vi "TSM Relay Publish Relay Operated.vi"(0 "TSM Relay in":T1={"TSM context"=refnum, "Pin Query Context"=refnum, "TSM Site Numbers"=[], "SSC Relay"=[], "Unfiltered Pins"=[], "Filtered Pins"=[], "Filtered Pins Info"={"Unfiltered Pins Count"=3, "Locations"=[], "Lengths"=[]}}, 1 "Published Data Id":string, 7 "Completed Relay Operations":T5[](array[typedef]) {"Desired State" items=["Open Relay"=20, "Close Relay"=21]}, 11 "error in":errorcluster) -> (4 "TSM Relay out":T1={"TSM context"=refnum, "Pin Query Context"=refnum, "TSM Site Numbers"=[], "SSC Relay"=[], "Unfiltered Pins"=[], "Filtered Pins"=[], "Filtered Pins Info"={"Unfiltered Pins Count"=3, "Locations"=[], "Lengths"=[]}}, 15 "error out":errorcluster)   [LabVIEW 2019]
doc: "This VI publishes the Relay Operated? information from each Relay in the TSM Relay session."
uses:
  SubVIs/TSM SSC Relay.ctl
  <vilib>/NI_TestStand_SemiconductorModule/NI_TestStand_Semiconductor_Module.lvlibp/PinMap/PinQueryContext/MultiplePinMultipleSessionQueryContext/MultiplePinMultipleSessionQueryContext.lvclass
  C:/Program Files/National Instruments/LabVIEW 2019/vi.lib/NI_TestStand_SemiconductorModule/NI_TestStand_Semiconductor_Module.lvlibp/PinMap/PinQueryContext/MultipleSessionPinQueryContext.lvclass
  <vilib>/NI_TestStand_SemiconductorModule/NI_TestStand_Semiconductor_Module.lvlibp/PinMap/General/SemiconductorModuleContext.ctl
  SSC/SSC Relay.ctl
  SubVIs/TSM Filtered Pins Info.ctl
  SubVIs/TSM Relay Completed Operations.ctl
  <instrlib>/niSwitch/niSwitch.llb/niSwitch Relay Action.ctl
  <vilib>/NI_TestStand_SemiconductorModule/NI_TestStand_Semiconductor_Module.lvlibp/PinMap/General/Publish/PublishDataDouble2D.vi
  <vilib>/NI_TestStand_SemiconductorModule/NI_TestStand_Semiconductor_Module.lvlibp
  C:/Program Files/National Instruments/LabVIEW 2019/vi.lib/NI_TestStand_SemiconductorModule/NI_TestStand_Semiconductor_Module.lvlibp/PinMap/PinQueryContext/PinQueryContext.lvclass
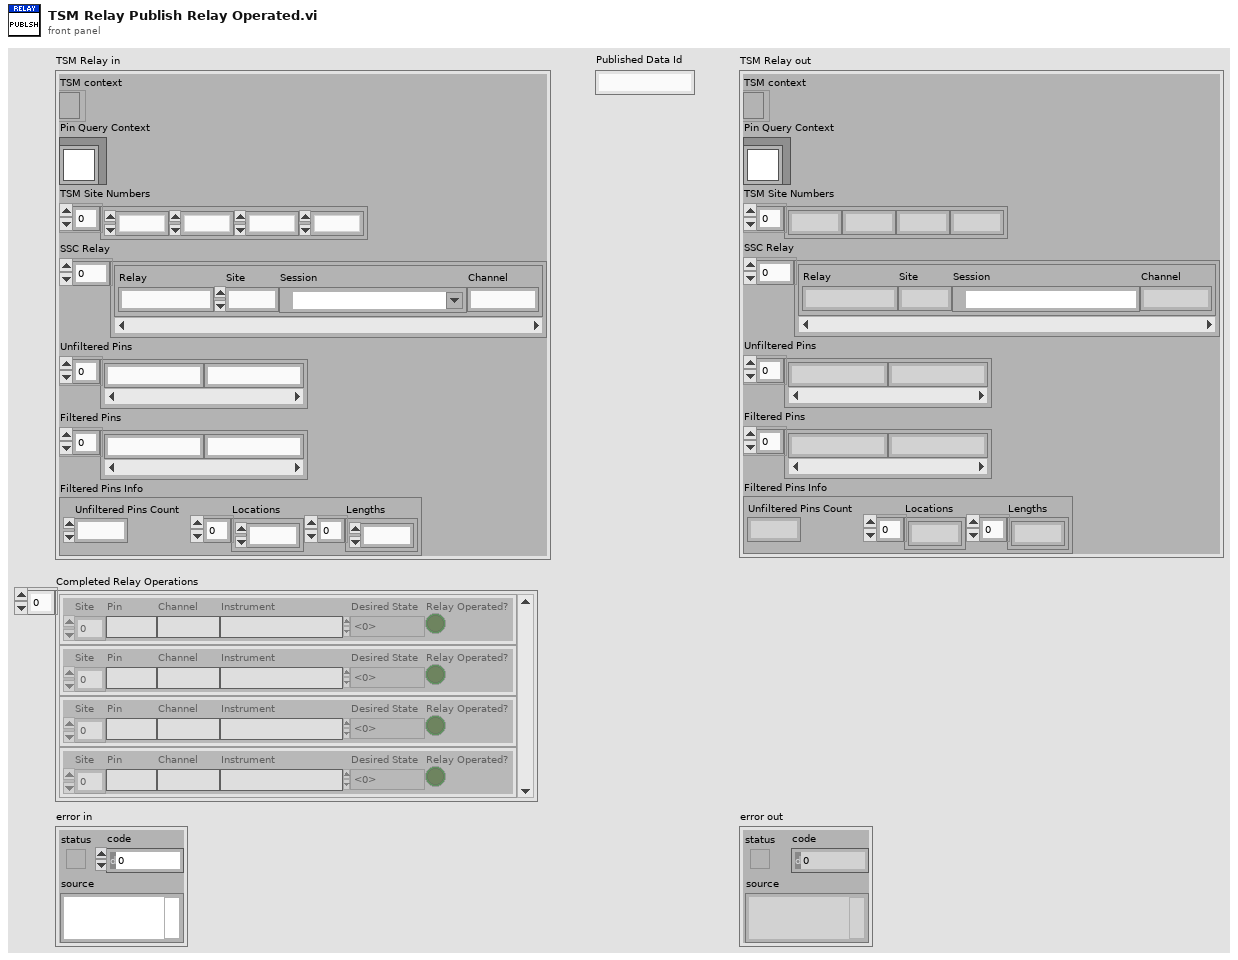
[diagram p1: front panel]
types:
  T1 = typedef "TSM SSC Relay.ctl" = cluster{"TSM context":T2, "Pin Query Context":refnum<class "MultiplePinMultipleSessionQueryContext.lvclass">, "TSM Site Numbers":i32[], "SSC Relay":T3[], "Unfiltered Pins":string[], "Filtered Pins":string[], "Filtered Pins Info":T4}
  T2 = typedef "NI_TestStand_Semiconductor_Module.lvlibp/SemiconductorModuleContext.ctl" = refnum<k7>
  T3 = typedef "SSC Relay.ctl" = cluster{"Relay":string, "Site":i32, "Session":refnum<k15>, "Channel":string}
  T4 = typedef "TSM Filtered Pins Info.ctl" = cluster{"Unfiltered Pins Count":i32, "Locations":i32[], "Lengths":i32[]}
  T5 = typedef "TSM Relay Completed Operations.ctl" = cluster{"Site":i32, "Pin":string, "Channel":string, "Instrument":string, "Desired State":T6, "Relay Operated?":bool}
  T6 = typedef "niSwitch Relay Action.ctl" = i32
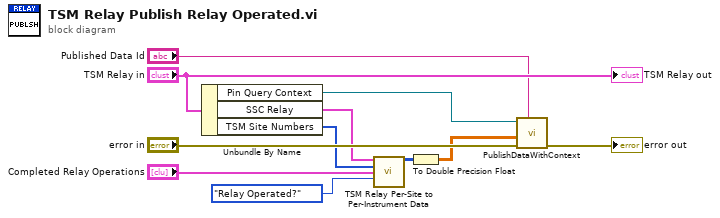
[diagram p0: block diagram]
diagram:
  n1 = Unbundle By Name("TSM Relay in") -> ("Pin Query Context"=w11:refnum<class "MultiplePinMultipleSessionQueryContext.lvclass">, "SSC Relay"=w5:T3[], "TSM Site Numbers"=w6:i32[])
  n2 = call "TSM Relay Per-Site to Per-Instrument Data.vi"("SSC Relay"=w5, "TSM Site Numbers"=w6, "Completed Relay Operations"="Completed Relay Operations", "Selection"=enum16{"Desired State", "Relay Operated?"}."Relay Operated?") -> ("Per-Instrument Per-Relay Data"=w1:i32[][])  [unwired: 11 in]
  n3 = To Double Precision Float(number=w1) -> (double precision float=w8:dbl[][])
  n4 = call-poly <vilib>:"PublishDataWithContext.vi"("Published Data Id"="Published Data Id", "error in (no error)"="error in", "Data In"=w8, "Pin Query Context"=w11) -> ("error out"=→"error out":errorcluster)  [unwired: 6 in, 1 out]
  "TSM Relay out" <- "TSM Relay in"
